vi "LCDoutput.vi"() -> ()   [LabVIEW 2011]
uses:
  <vilib>/EmbeddedDisplay/Hitachi HD44780/FPGA/Internal/LCD Command.vi
  <vilib>/EmbeddedDisplay/Hitachi HD44780/FPGA/Public/Command Handler (8 Bits).vi
  <vilib>/eio/EIONode/EIONode.xnode
  <vilib>/rvi/eio/common/nirviEmuTemplateMethod_errors.vi
  <vilib>/EmbeddedDisplay/Hitachi HD44780/FPGA/HD44780 FPGA.lvlib
panel:
  in  "LCD Command":T1={"device index (-1)"=-1, "operation (0)"=0}
  in  "stop":bool
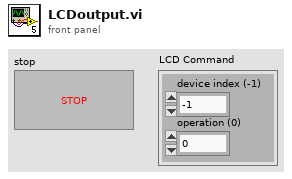
[diagram p1: front panel]
types:
  T1 = cluster{"device index (-1)":i8, "operation (0)":u32}
  T2 = enum8{"increment & no shift", "increment & shift", "decrement & no shift", "decrement & shift"}
  T3 = cluster{"RS":refnum<k21>, "R/W":refnum<k21>, "E1":refnum<k21>, "E2":refnum<k21>, "DB0":refnum<k21>, "DB1":refnum<k21>, "DB2":refnum<k21>, "DB3":refnum<k21>, "DB4":refnum<k21>, "DB5":refnum<k21>, "DB6":refnum<k21>, "DB7":refnum<k21>}
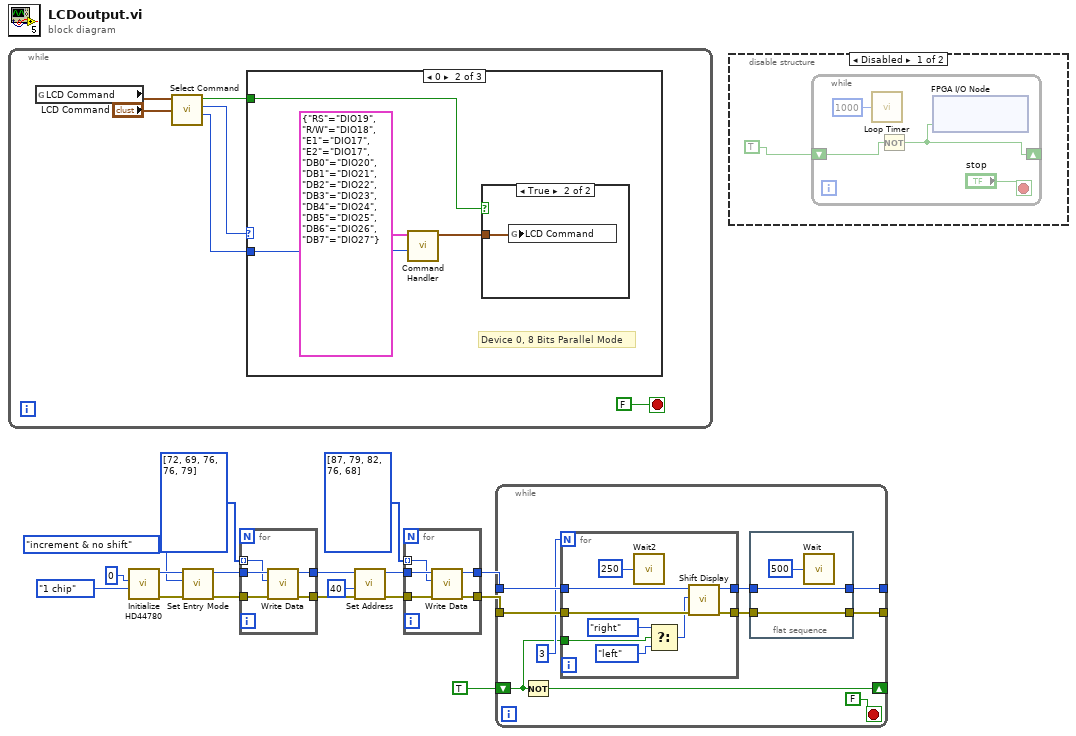
[diagram p0: block diagram]
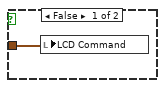
[diagram p3: hidden frame]
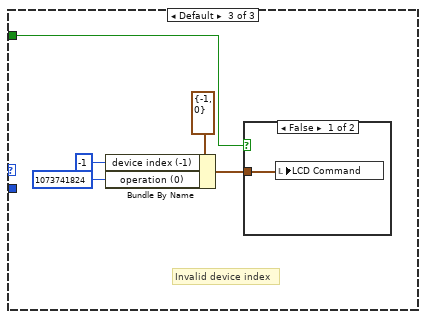
[diagram p4: hidden frame]
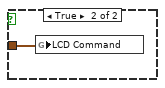
[diagram p5: hidden frame]
diagram:
  n1 = while {
    stop <- FALSE stop-if-true
    n2 = global read "LCD Command.vi" "LCD Command"() -> (w18:T1)
    n3 = call <vilib>:"Select Command.vi"("Host LCD Command"="LCD Command", "FPGA LCD Command"=w18) -> ("operation"=w20:u32, "device index"=w21:i8, "FPGA? True : False"=w19:bool)  [unwired: 7 in]
    n4 = case shown="0" w21 {
      tunnel: w20 -> [_ w27 _]
      tunnel: w19 -> [_ w26 w34]
      frame -1 {
        # "IDLE State"
      }
      frame 0 {
        # "Device 0, 8 Bits Parallel Mode"
        n5 = call-poly <vilib>:"Command Handler.vi"("operation"=w27, "device connection map in"=T3 {"RS"="DIO19", "R/W"="DIO18", "E1"="DIO17", "E2"="DIO17", "DB0"="DIO20", "DB1"="DIO21", "DB2"="DIO22", "DB3"="DIO23", "DB4"="DIO24", "DB5"="DIO25", "DB6"="DIO26", "DB7"="DIO27"}) -> ("result"=w25:T1)  [unwired: 9 in]
        n6 = case shown="True" w26 {
          tunnel: w25 -> [w28 w29]
          frame False {
            n7 = local write "LCD Command"(w28) -> ()
          }
          frame True {
            n8 = global write "LCD Command.vi" "LCD Command"(w29) -> ()
          }
        }
      }
      frame Default {
        # "Invalid device index"
        n9 = Bundle By Name(cluster=T1 {"device index (-1)"=-1, "operation (0)"=0} ("LCD Command"), "device index (-1)"=i8 -1 ("LCD_device index (-1)"), "operation (0)"=u32 1073741824 ("LCD_operation (0)")) -> (w30:T1)
        n10 = case shown="False" w34 {
          tunnel: w30 -> [w35 w36]
          frame False {
            n11 = local write "LCD Command"(w35) -> ()
          }
          frame True {
            n12 = global write "LCD Command.vi" "LCD Command"(w36) -> ()
          }
        }
      }
    }
  }
  n13 = call <vilib>:"Initialize HD44780.vi"("number of chips"=enum8{"1 chip", "2 chips"}."1 chip", "device index"=i8 0) -> ("error out"=w13:errorcluster, "LCD out"=w15:u32)  [unwired: 8 in]
  n14 = call <vilib>:"Set Entry Mode.vi"("error in (no error)"=w13, "entry mode"=T2."increment & no shift", "LCD in"=w15) -> ("error out"=w12:errorcluster, "LCD out"=w14:u32)  [unwired: 7 in]
  n15 = for {
    tunnel: w14 -> [w41]
    tunnel: w12 -> [w40]
    tunnel: u8[] [72, 69, 76, 76, 79] -> [w39] mode=indexing
    tunnel: [w38] -> w9
    tunnel: [w37] -> w10
    n16 = call <vilib>:"Write Data.vi"("error in (no error)"=w40, "character code"=w39, "LCD in"=w41) -> ("error out"=w38:errorcluster, "LCD out"=w37:u32)  [unwired: 7 in]
  }
  n17 = call <vilib>:"Set Address.vi"("error in (no error)"=w9, "address"=u8 40, "LCD in"=w10) -> ("error out"=w3:errorcluster, "LCD out"=w4:u32)  [unwired: 7 in]
  n18 = for {
    tunnel: w4 -> [w46]
    tunnel: w3 -> [w45]
    tunnel: u8[] [87, 79, 82, 76, 68] -> [w44] mode=indexing
    tunnel: [w43] -> w2
    tunnel: [w42] -> w5
    n19 = call <vilib>:"Write Data.vi"("error in (no error)"=w45, "character code"=w44, "LCD in"=w46) -> ("error out"=w43:errorcluster, "LCD out"=w42:u32)  [unwired: 7 in]
  }
  n20 = while {
    tunnel: w5 -> [w55]
    tunnel: w2 -> [w54]
    shift-right: [w51] -> _
    shift-left: TRUE -> [w52]
    tunnel: [w49] -> _
    tunnel: [w47] -> _
    stop <- FALSE stop-if-true
    n21 = Not(x=w52) -> (.not. x?=w51:bool)
    n22 = for {
      N: 3 -> [_]
      tunnel: [w68] -> w50
      tunnel: [w67] -> w48
      tunnel: w55 -> [w66]
      tunnel: w54 -> [w65]
      tunnel: w52 -> [w60]
      n23 = call "Wait2"("Count(mSec)"=u32 250) -> ()  [unwired: 1 out]
      n24 = Select(t=enum16{"left", "right"}."right" ("direction"), s=w60, f=enum16{"left", "right"}."left" ("direction")) -> (s? t:f=w62:enum16{"left", "right"})
      n25 = call <vilib>:"Shift Display.vi"("error in (no error)"=w65, "direction"=w62, "LCD in"=w66) -> ("error out"=w67:errorcluster, "LCD out"=w68:u32)  [unwired: 7 in]
    }
    n26 = flat-sequence {
      tunnel: w50 -> [w58]
      tunnel: [w58] -> w49
      tunnel: w48 -> [w57]
      tunnel: [w57] -> w47
      frame #0 {
        n27 = call "Wait"("Count(mSec)"=u32 500) -> ()  [unwired: 1 out]
      }
    }
  }
  n28 = disable-structure shown="Disabled" {
    frame Disabled {
      n29 = while {
        shift-right: [w71] -> _
        shift-left: TRUE -> [w73]
        stop <- "stop" stop-if-true
        n30 = call "Loop Timer"("Count(mSec)"=u32 1000 ("Count(Ticks)")) -> ()  [unwired: 1 out]
        n31 = Not(x=w73) -> (.not. x?=w71:bool)
        n32 = xnode "FPGA I/O Node"("FPGA LED"=w71) -> ()  [unwired: 1 in, 1 out]
      }
    }
    frame Enabled {
    }
  }
